vi "Read Parent Attributes.vi"(11 "Actor in":refnum<class "Actor.lvclass">) -> (2 "Parent Attributes":refnum<data-value>)   [LabVIEW 2020, in "jettl.lvlib" / "Actor.lvclass"]
uses:
  Actor.lvclass
  Msg/Msg.lvclass
  Transport/Transport.lvclass
  Actor Attributes.ctl
  jettl.lvlib
  Msgs.ctl
  Msg Names.ctl
  Unified Layer.ctl
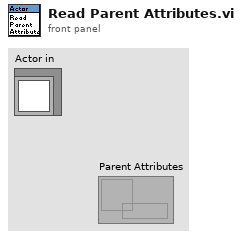
[diagram p1: front panel]
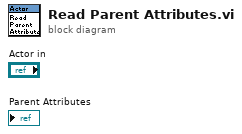
[diagram p0: block diagram]
diagram:
